vi "test_generic.vi"() -> ()   [LabVIEW 2010, in "GenericExperimentController.lvclass"]
uses:
  GenericExperimentController.lvclass
  main/labview_source/type_definitions/clusters/controls_refs.ctl
  trigger_enum.ctl
  common/classes/GenericComponent/GenericComponent/GenericComponent.lvclass
panel:
  in  "create and send":bool
  in  "proceed button":bool
  in  "stop":bool
  in  "scan start button":bool
  # "Test GenericExperimentController"
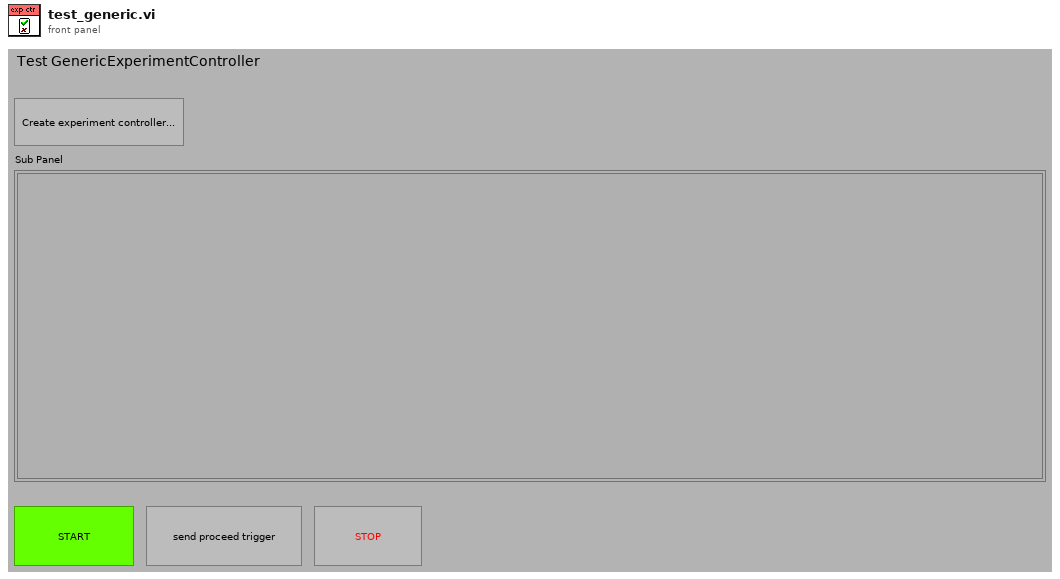
[diagram p1: front panel]
types:
  T1 = typedef "controls_refs.ctl" = cluster{"scan start button":refnum<vi>, "tabs":cluster{"main":refnum<vi>, "settings":refnum<vi>}, "subpanels":cluster{"imagingMode":refnum<vi>, "scanHead":refnum<vi>, "display":refnum<vi>, "experimentController":refnum<vi>, "instrument":refnum<vi>, "stage":refnum<vi>, "stimulator":refnum<vi>, "dataCollection":refnum<vi>, "analyser":refnum<vi>, "daq":refnum<vi>, "imageAssembler":refnum<vi>}, "drop-downs":cluster{"run mode":refnum<vi>, "imagingMode":refnum<vi>, "experimentalController":refnum<vi>, "objective":refnum<vi>}, "status lights":cluster{"experimentController":refnum<vi>, "imagingMode":refnum<vi>, "scanHead":refnum<vi>, "daq":refnum<vi>, "imageAssembler":refnum<vi>, "dataCollection":refnum<vi>, "display":refnum<vi>, "analyser":refnum<vi>, "stage":refnum<vi>, "stimulator":refnum<vi>, "instrument":refnum<vi>}, "message":refnum<vi>, "stimulator enabled?":refnum<vi>, "saving":cluster{"data folder path":refnum<vi>, "file base name":refnum<vi>, "notebook":refnum<vi>}, "progress bar":refnum<vi>, "update icon":refnum<vi>, "title":refnum<vi>, "main vi":refnum<vi>, "user":refnum<vi>, "exit_button":refnum<vi>, "CPU usage %":refnum<vi>}
  T2 = typedef "GenericExperimentController.lvclass/trigger_enum.ctl" = enum16{"NULL", "initialise", "terminate", "start", "stop", "proceed", "prepare"}
  T3 = typedef "XComponentSpecification.xctl/data.ctl" = cluster{"class path":string, "configuration":string, "label":string, "settings name":string}
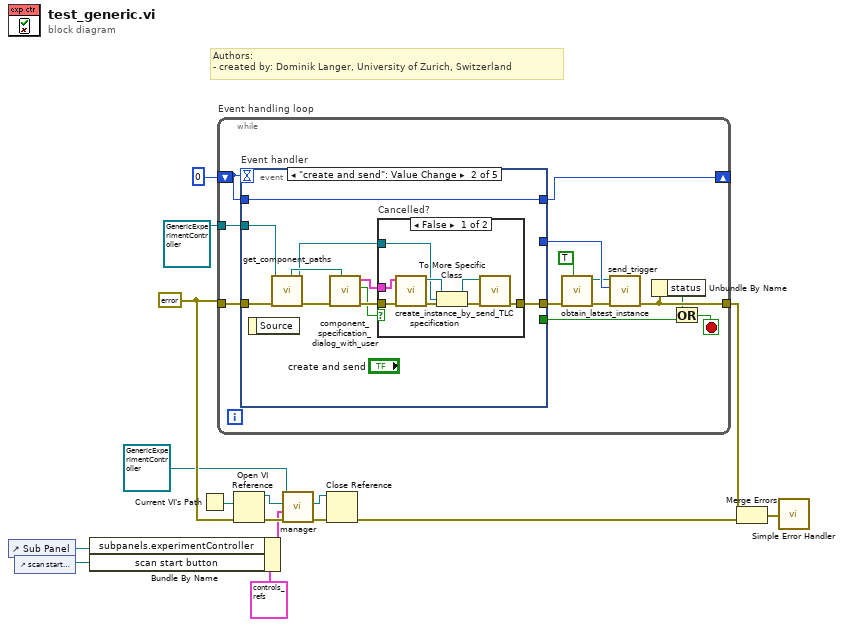
[diagram p0: block diagram]
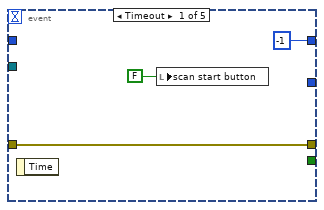
[diagram p2: hidden frame]
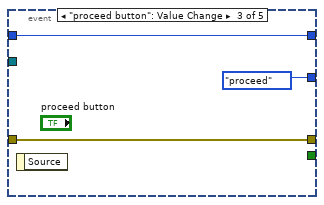
[diagram p4: hidden frame]
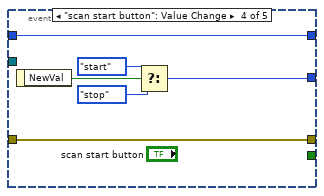
[diagram p5: hidden frame]
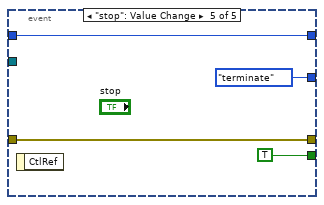
[diagram p6: hidden frame]
diagram:
  w9 = errorcluster {"status"=FALSE, "code"=0, "source"=""} ("error out")
  # "Authors: \n- created by: Dominik Langer, University of Zurich, Switzerland"
  n1 = control-ref of="Sub Panel"() -> (w15:refnum<vi>)
  n2 = control-ref of="scan start button"() -> (w11:refnum<vi>)
  n3 = Bundle By Name(cluster=T1 {"scan start button"=refnum, "tabs"={"main"=refnum, "settings"=refnum}, "subpanels"={"imagingMode"=refnum, "scanHead"=refnum, "display"=refnum, "experimentController"=refnum, "instrument"=refnum, "stage"=refnum, "stimulator"=refnum, "dataCollection"=refnum, "analyser"=refnum, "daq"=refnum, "imageAssembler"=refnum}, "drop-downs"={"run mode"=refnum, "imagingMode"=refnum, "experimentalController"=refnum, "objective"=refnum}, "status lights"={"experimentController"=refnum, "imagingMode"=refnum, "scanHead"=refnum, "daq"=refnum, "imageAssembler"=refnum, "dataCollection"=refnum, "display"=refnum, "analyser"=refnum, "stage"=refnum, "stimulator"=refnum, "instrument"=refnum}, "message"=refnum, "stimulator enabled?"=refnum, "saving"={"data folder path"=refnum, "file base name"=refnum, "notebook"=refnum}, "progress bar"=refnum, "update icon"=refnum, "title"=refnum, "main vi"=refnum, "user"=refnum, "exit_button"=refnum, "CPU usage %"=refnum} ("control references"), "subpanels.experimentController"=w15, "scan start button"=w11) -> (w2:T1)
  n4 = Current VI's Path() -> (path=w10:path)
  n5 = while "Event handling loop" {
    shift-right: [w26] -> _
    shift-left: 0 -> [w27]
    tunnel: refnum<class "GenericExperimentController.lvclass"> refnum ("GenericExperimentController.lvclass") -> [w21]
    tunnel: w9 -> [w29]
    tunnel: [w20] -> w14
    stop <- w17 stop-if-true
    n6 = event "Event handler" shown="[1] \"create and send\": Value Change" {
      selector: _ -> [_ _ _ _ _]
      dyn-events: _ -> [_ _ _ _ _]
      timeout: w27 -> [_ _ _ _ _]
      tunnel: [w30 w41 w54 w60 w64] -> w25
      tunnel: w29 -> [w30 w39 w54 w60 w64]
      tunnel: [_ _ trigger_enum."proceed" ("trigger") w56 trigger_enum."terminate" ("trigger")] -> w28
      tunnel: [_ _ _ _ TRUE] -> w19
      tunnel: [-1 w42 w53 w55 w61] -> w26
      tunnel: w27 -> [_ w42 w53 w55 w61]
      tunnel: w21 -> [_ w36 _ _ _]
      event Timeout {
        n7 = event-data() -> ()  [unwired: 2 out]
        n8 = local write "scan start button"(FALSE ("scan start button")) -> ()
      }
      event "create and send": Value Change {
        n9 = event-data() -> ()  [unwired: 2 out]
        n10 = call-dynamic "get_component_paths.vi"("error in (no error)"=w39, "GenericComponent in"=w36) -> ("error out"=w40:errorcluster, "GenericComponent out"=w35:refnum<class "GenericExperimentController.lvclass">, "component type directory"=w37:path)  [unwired: 4 in, 3 out]
        n11 = call "component_specification_dialog_with_user.vi"("start path"=w37, "error in (no error)"=w40) -> ("error out"=w38:errorcluster, "cancelled?"=w34:bool, "component specification out"=w33:T3)  [unwired: 7 in]
        n12 = case "Cancelled?" shown="False" w34 {
          tunnel: [w50 w51] -> w41
          tunnel: w38 -> [w45 w51]
          tunnel: w35 -> [w44 _]
          tunnel: w33 -> [w43 _]
          frame False {
            n13 = call "create_instance_by_specification.vi"("error in (no error)"=w45, "component specification"=w43) -> ("error out"=w47:errorcluster, "GenericPlugin out"=w46:refnum<class "GenericComponent.lvclass">)  [unwired: 7 in, 1 out]
            n14 = To More Specific Class(target class=w44, reference=w46, error in=w47) -> (specific class reference=w48:refnum<class "GenericExperimentController.lvclass">, error out=w49:errorcluster)
            n15 = call-dynamic "send_TLC.vi"("error in (no error)"=w49, "GenericExperimentController in"=w48) -> ("error out"=w50:errorcluster)  [unwired: 9 out]
          }
          frame True {
          }
        }
      }
      event "proceed button": Value Change {
        n16 = event-data() -> ()  [unwired: 2 out]
      }
      event "scan start button": Value Change {
        n17 = event-data() -> ("NewVal"=w58:bool)  [unwired: 1 out]
        n18 = Select(t=trigger_enum."start" ("trigger"), s=w58, f=trigger_enum."stop" ("trigger")) -> (s? t:f=w56:T2)
      }
      event "stop": Value Change {
        n19 = event-data() -> ()  [unwired: 2 out]
      }
    }
    n20 = call "obtain_latest_instance.vi"("quick, but maybe outdated?"=TRUE, "error in (no error)"=w25) -> ("error out"=w24:errorcluster, "GenericExperimentController out"=w23:refnum<class "GenericExperimentController.lvclass">)  [unwired: 8 out]
    n21 = call-dynamic "send_trigger.vi"("error in (no error)"=w24, "trigger"=w28, "GenericExperiment in"=w23) -> ("error out"=w20:errorcluster)  [unwired: 8 out]
    n22 = Unbundle By Name(w20) -> ("status"=w18:bool)
    n23 = Or(x=w18, y=w19) -> (x .or. y?=w17:bool)
  }
  n24 = Open VI Reference(vi path=w10, error in (no error)=w9) -> (vi reference=w4:refnum<vi>, error out=w6:errorcluster)  [unwired: 4 out]
  n25 = call-dynamic "manager.vi"("error in (no error)"=w6, "control references"=w2, "top-level VI ref in"=w4, "GenericToplevelComponent in"=refnum<class "GenericExperimentController.lvclass"> refnum ("GenericExperimentController.lvclass")) -> ("error out"=w5:errorcluster, "top-level VI ref out"=w3:refnum<vi>)  [unwired: 5 in, 1 out]
  n26 = Close Reference(reference=w3, error in (no error)=w5) -> (error out=w8:errorcluster)
  n27 = Merge Errors(w14, w8) -> (w13:errorcluster)
  n28 = call <vilib>:"Simple Error Handler.vi"("error in (no error)"=w13) -> ()  [unwired: 1 in, 8 out]
